vi "题目3.vi"() -> ()   [LabVIEW 2017]
uses:
  <vilib>/measure/NI_MABase.lvlib
panel:
  in  "基路径":path
  out "Y":dbl[](array[numeric])
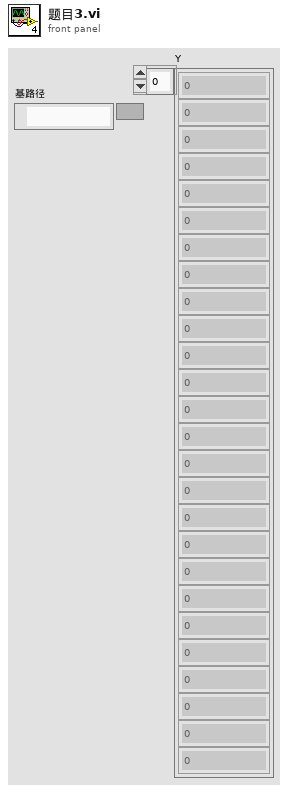
[diagram p1: front panel]
types:
  T1 = enum16{"open", "replace", "create", "open or create", "replace or create", "replace or create with confirmation"}
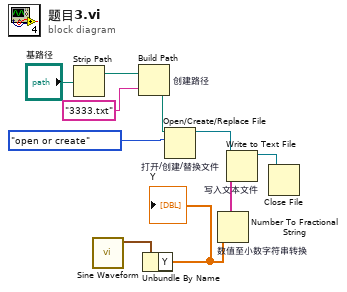
[diagram p0: block diagram]
diagram:
  n1 = Strip Path(path="基路径") -> (stripped path=w4:path)  [unwired: 1 out]
  n2 = call <vilib>:"Sine Waveform.vi"() -> ("signal out"=w10:waveform(dbl))  [unwired: 10 in, 1 out]
  n3 = Build Path "创建路径"(base path=w4, name or relative path="3333.txt" ("名称或相对路径")) -> (appended path=w6:path)
  n4 = Unbundle By Name(w10) -> ("Y"=w1:dbl[])
  "Y" <- w1
  n5 = Open/Create/Replace File "打开/创建/替换文件"(file path (use dialog)=w6, operation (0:open)=T1."open or create" ("操作(0:open)")) -> (refnum out=w8:refnum<file>)  [unwired: 4 in, 2 out]
  n6 = Number To Fractional String "数值至小数字符串转换"(number=w1) -> (F-format string=w9:string[])  [unwired: 3 in]
  n7 = Write to Text File "写入文本文件"(file (use dialog)=w8, text=w9) -> (refnum out=w7:refnum<file>)  [unwired: 2 in, 2 out]
  n8 = Close File(refnum=w7) -> ()  [unwired: 1 in, 2 out]
